vi "BRig_Host_dataRunState__entryAdd_v3.vi"(0 "input_dataPlot":u16[][](array[numeric]), 1 "input_dataTS":u16[][](array[numeric]), 2 "input_idx":i32[](array[numeric]), 4 "input_nTrial":u16, 5 "input_LorR":u16, 7 "input_sSelection":u16, 8 "input_trig_l2":u16, 9 "input_tSelection":u16, 10 "input_trig_l1":u16, 11 "input_tSelectionPlot":u16, 13 "input_iSelection":u16) -> (14 "output_dataPlot":u16[][](array[numeric]), 15 "output_dataTS":u16[][](array[numeric]), 16 "output_idx":i32[](array[numeric]), 18 "output_updatePlot":bool)   [LabVIEW 2014]
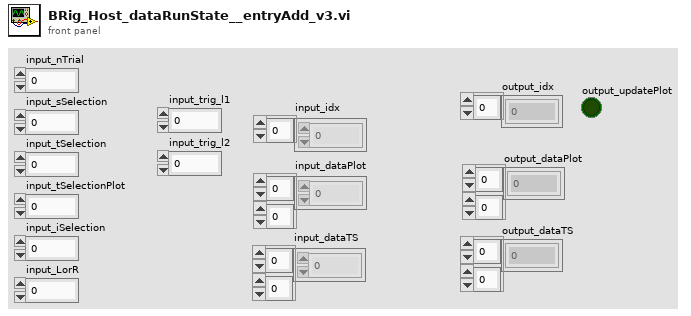
[diagram p1: front panel]
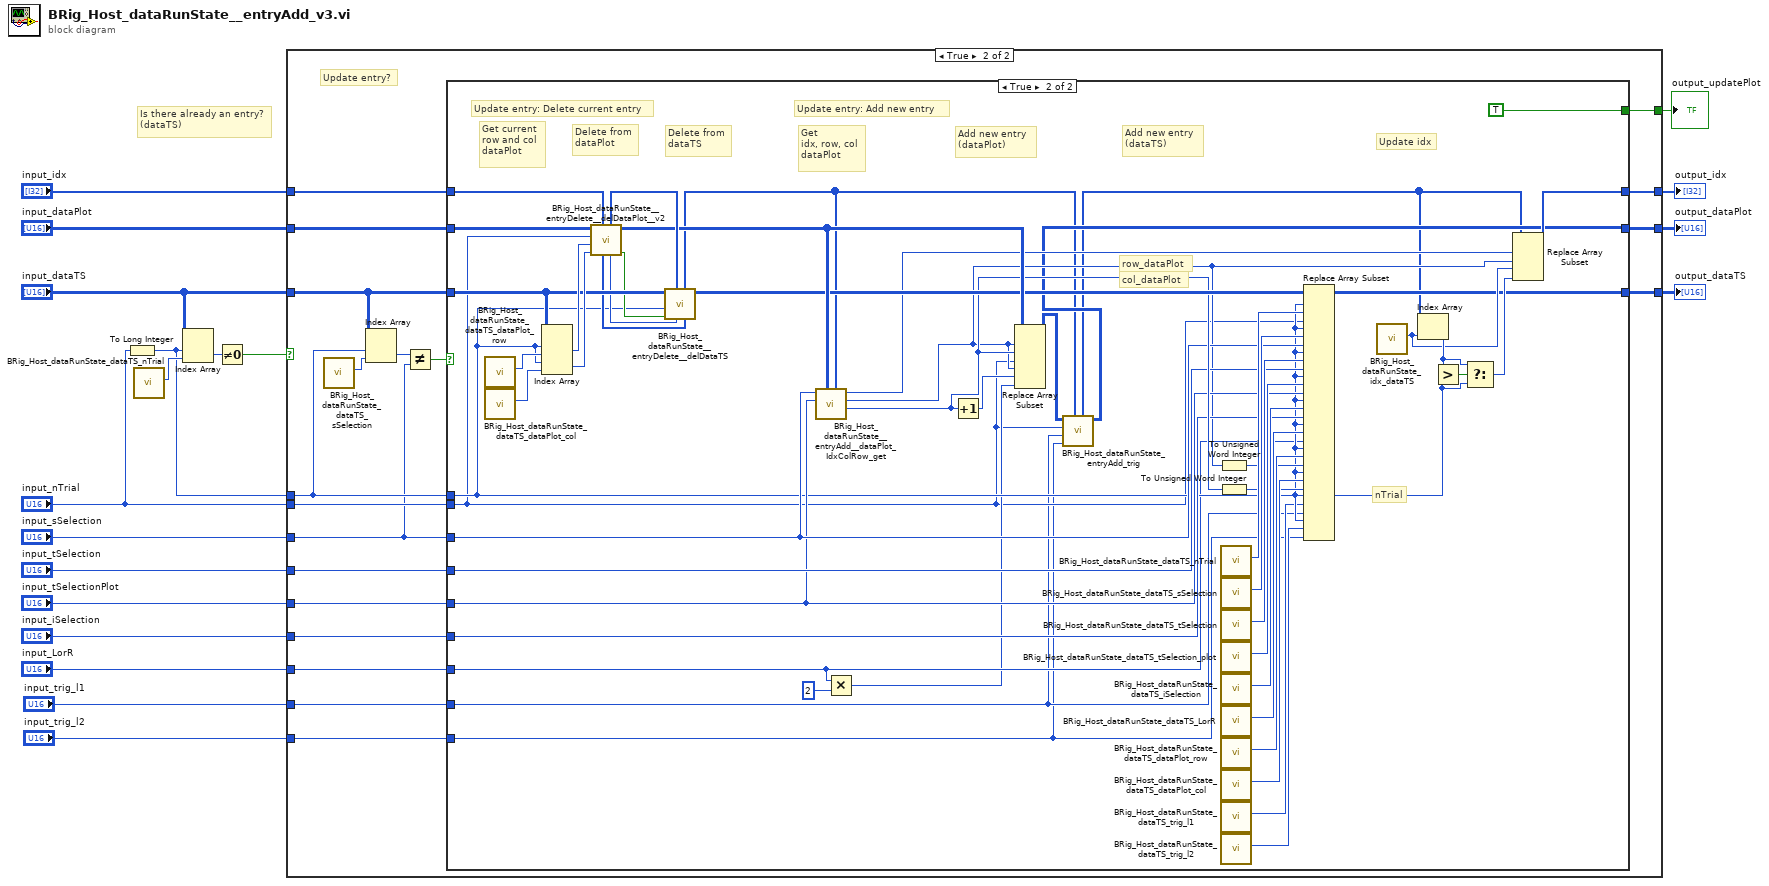
[diagram p0: block diagram]
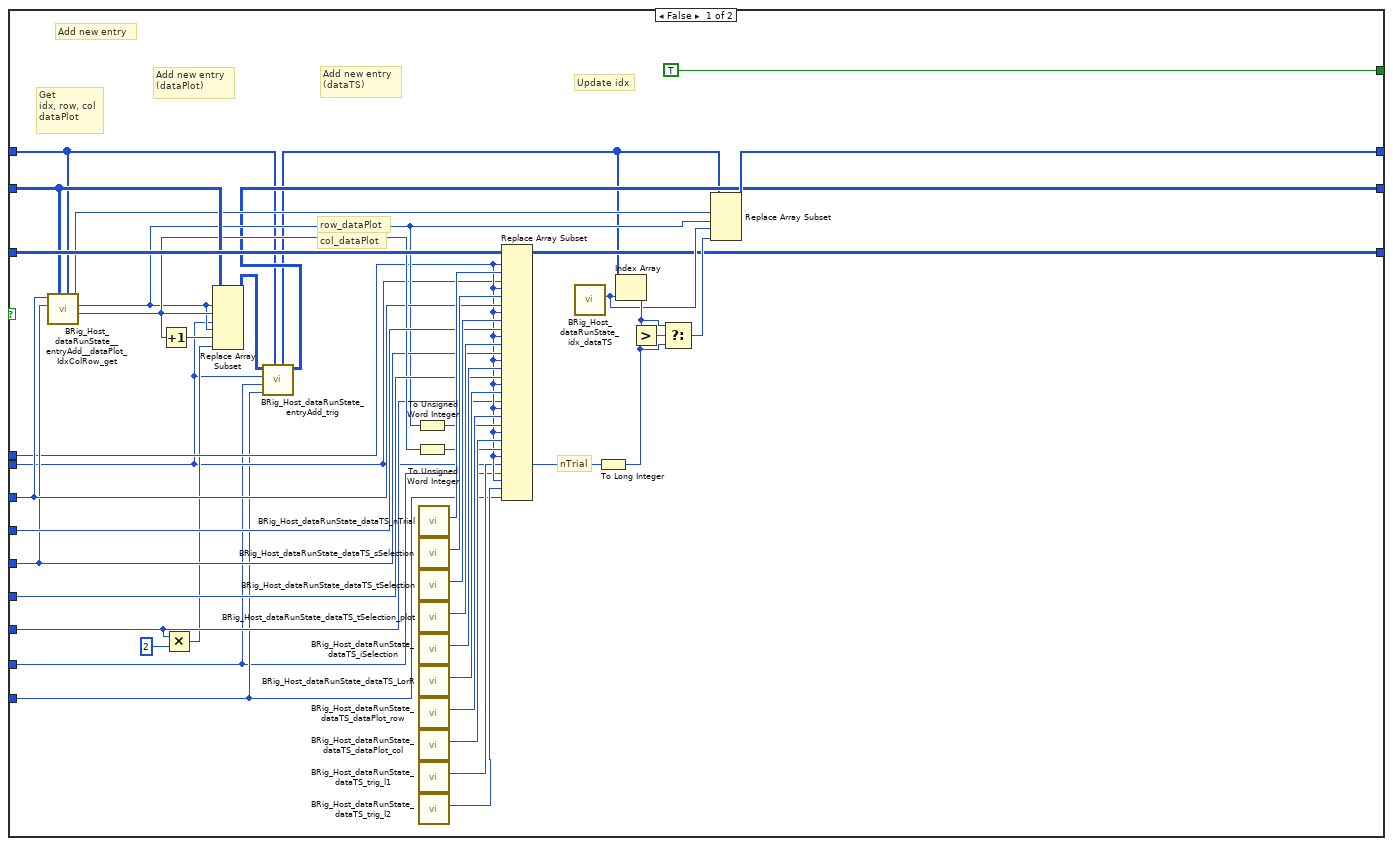
[diagram p2: hidden frame]
diagram:
  # "Is there already an entry?\n(dataTS)"
  n1 = To Long Integer(number="input_nTrial") -> (32bit integer=w15:i32)
  n2 = call "BRig_Host_dataRunState_dataTS_nTrial.vi"() -> ("output_idx_dataTS_nTrial"=w19:i32)  [unwired: 11 in]
  n3 = Index Array(array="input_dataTS", index (row)=w15, index (col)=w19) -> (element=w18:u16)
  n4 = Not Equal To 0?(x=w18) -> (x != 0?=w17:bool)
  n5 = case shown="True" w17 {
    tunnel: "input_nTrial" -> [w22 w69]
    tunnel: w15 -> [w31 w71]
    tunnel: "input_dataTS" -> [w60 w73]
    tunnel: "input_idx" -> [w24 w77]
    tunnel: "input_dataPlot" -> [w38 w75]
    tunnel: "input_sSelection" -> [w35 w63]
    tunnel: "input_tSelectionPlot" -> [w34 w70]
    tunnel: "input_iSelection" -> [w48 w66]
    tunnel: "input_LorR" -> [w28 w68]
    tunnel: [w50 w76] -> w6
    tunnel: [w25 w74] -> w5
    tunnel: [w43 w72] -> w4
    tunnel: "input_tSelection" -> [w49 w67]
    tunnel: [TRUE w65] -> w3
    tunnel: "input_trig_l1" -> [w20 w62]
    tunnel: "input_trig_l2" -> [w21 w61]
    frame False {
      # "Get\nidx, row, col\ndataPlot"
      # "nTrial"
      # "row_dataPlot"
      # "col_dataPlot"
      # "Update idx"
      # "Add new entry\n(dataPlot)"
      # "Add new entry"
      # "Add new entry\n(dataTS)"
      n6 = call "BRig_Host_dataRunState__entryAdd__dataPlot_IdxColRow_get.vi"("input_idx"=w24, "input_dataPlot"=w38, "input_tSelectionPlot"=w34, "input_sSelection"=w35) -> ("output_col_dataPlot"=w36:i32, "output_row_dataPlot"=w33:i32, "output_idx_dataPlot"=w37:i32)  [unwired: 5 in]
      n7 = Increment(x=w36) -> (x+1=w51:i32)
      n8 = Multiply(x=w28, y=u16 2) -> (x*y=w27:u16)
      n9 = Replace Array Subset(array=w38, new element #1=w22, index (row) #1=w33, index (col) #1=w36, new element #2=w27, index (row) #2=w33, index (col) #2=w51) -> (w26:u16[][])
      n10 = call "BRig_Host_dataRunState_entryAdd_trig.vi"("input_idx"=w24, "input_trig_l2"=w21, "input_trig_l1"=w20, "input_nTrial"=w22, "input_dataPlot"=w26) -> ("output_dataPlot"=w25:u16[][], "output_idx"=w23:i32[])  [unwired: 5 in]
      n11 = To Unsigned Word Integer(number=w33) -> (unsigned 16bit integer=w42:u16)
      n12 = To Unsigned Word Integer(number=w36) -> (unsigned 16bit integer=w41:u16)
      n13 = call "BRig_Host_dataRunState_dataTS_nTrial.vi"() -> ("output_idx_dataTS_nTrial"=w59:i32)  [unwired: 11 in]
      n14 = call "BRig_Host_dataRunState_dataTS_sSelection.vi"() -> ("output_idx_dataTS_sSelection"=w58:i32)  [unwired: 11 in]
      n15 = call "BRig_Host_dataRunState_dataTS_tSelection.vi"() -> ("output_idx_dataTS_tSelection"=w57:i32)  [unwired: 11 in]
      n16 = call "BRig_Host_dataRunState_dataTS_tSelection_plot.vi"() -> ("output_idx_dataTS_tSelection_plot"=w56:i32)  [unwired: 11 in]
      n17 = call "BRig_Host_dataRunState_dataTS_iSelection.vi"() -> ("output_idx_dataTS_iSelection"=w55:i32)  [unwired: 11 in]
      n18 = call "BRig_Host_dataRunState_dataTS_LorR.vi"() -> ("output_idx_dataTS_LorR"=w54:i32)  [unwired: 11 in]
      n19 = call "BRig_Host_dataRunState_dataTS_dataPlot_row.vi"() -> ("output_idx_dataTS_dataPlot_row"=w53:i32)  [unwired: 11 in]
      n20 = call "BRig_Host_dataRunState_dataTS_dataPlot_col.vi"() -> ("output_idx_dataTS_dataPlot_col"=w52:i32)  [unwired: 11 in]
      n21 = call "BRig_Host_dataRunState_dataTS_trig_l1.vi"() -> ("output_idx_dataTS_trig_l1"=w30:i32)  [unwired: 11 in]
      n22 = call "BRig_Host_dataRunState_dataTS_trig_l2.vi"() -> ("output_idx_dataTS_trig_l2"=w29:i32)  [unwired: 11 in]
      n23 = Replace Array Subset(array=w60, new element #1=w22, index (row) #1=w31, index (col) #1=w59, new element #2=w35, index (row) #2=w31, index (col) #2=w58, new element #3=w49, index (row) #3=w31, index (col) #3=w57, new element #4=w34, index (row) #4=w31, index (col) #4=w56, new element #5=w48, index (row) #5=w31, index (col) #5=w55, new element #6=w28, index (row) #6=w31, index (col) #6=w54, new element #7=w42, index (row) #7=w31, index (col) #7=w53, new element #8=w41, index (row) #8=w31, index (col) #8=w52, new element #9=w20, index (row) #9=w31, index (col) #9=w30, new element #10=w21, index (row) #10=w31, index (col) #10=w29) -> (w43:u16[][])
      n24 = call "BRig_Host_dataRunState_idx_dataTS.vi"() -> ("output_idx_dataTS"=w45:i32)  [unwired: 11 in]
      n25 = To Long Integer(number=w22) -> (32bit integer=w40:i32)
      n26 = Index Array(array=w23, index=w45) -> (element=w46:i32)
      n27 = Greater?(x=w46, y=w40) -> (0:w47:bool)
      n28 = Select(t=w46, s=w47, f=w40) -> (s? t:f=w44:i32)
      n29 = Replace Array Subset(array=w23, new element #1=w33, index #1=w37, new element #2=w44, index #2=w45) -> (w50:i32[])
    }
    frame True {
      # "Update entry?"
      n30 = call "BRig_Host_dataRunState_dataTS_sSelection.vi"() -> ("output_idx_dataTS_sSelection"=w64:i32)  [unwired: 11 in]
      n31 = Index Array(array=w73, index (row)=w71, index (col)=w64) -> (element=w79:u16)
      n32 = Not Equal?(x=w79, y=w63) -> (x != y?=w78:bool)
      n33 = case shown="True" w78 {
        tunnel: w77 -> [w82 w128]
        tunnel: [w82 w107] -> w76
        tunnel: w75 -> [w81 w131]
        tunnel: [w81 w88] -> w74
        tunnel: w73 -> [w80 w127]
        tunnel: [w80 w104] -> w72
        tunnel: w71 -> [_ w95]
        tunnel: w63 -> [_ w101]
        tunnel: w70 -> [_ w99]
        tunnel: w69 -> [_ w87]
        tunnel: w68 -> [_ w91]
        tunnel: w67 -> [_ w100]
        tunnel: w66 -> [_ w98]
        tunnel: [_ TRUE] -> w65
        tunnel: w62 -> [_ w86]
        tunnel: w61 -> [_ w85]
        frame False {
          # "Do nothing"
        }
        frame True {
          # "nTrial"
          # "row_dataPlot"
          # "col_dataPlot"
          # "Update idx"
          # "Add new entry\n(dataPlot)"
          # "Add new entry\n(dataTS)"
          # "Get\nidx, row, col\ndataPlot"
          # "Update entry: Add new entry"
          # "Delete from\ndataTS"
          # "Delete from\ndataPlot"
          # "Get current\nrow and col\ndataPlot"
          # "Update entry: Delete current entry"
          n34 = call "BRig_Host_dataRunState_dataTS_dataPlot_row.vi"() -> ("output_idx_dataTS_dataPlot_row"=w133:i32)  [unwired: 11 in]
          n35 = call "BRig_Host_dataRunState_dataTS_dataPlot_col.vi"() -> ("output_idx_dataTS_dataPlot_col"=w132:i32)  [unwired: 11 in]
          n36 = Index Array(array=w127, index (row) #1=w95, index (col) #1=w133, index (row) #2=w95, index (col) #2=w132) -> (element #1=w129:u16, element #2=w130:u16)
          n37 = call "BRig_Host_dataRunState__entryDelete__delDataPlot__v2.vi"("input_idx"=w128, "input_col_dataPlot"=w130, "input_row_dataPlot"=w129, "input_nTrial"=w87, "input_dataPlot"=w131) -> (0:"output_arrTrials"=w125:bool, "output_dataPlot"=w106:u16[][], "output_arrTrials_length"=w124:i32, "output_idx"=w126:i32[], 6:"output_arrTrials"=w123:i32[])  [unwired: 2 in]
          n38 = call "BRig_Host_dataRunState__entryDelete__delDataTS.vi"(4:"output_arrTrials"=w123, "output_arrTrials_length"=w124, "input_idx"=w126, 8:"output_arrTrials"=w125, "input_nTrial"=w95, "input_dataTS"=w127) -> ("output_dataTS"=w105:u16[][], "output_idx"=w84:i32[])  [unwired: 4 in]
          n39 = call "BRig_Host_dataRunState__entryAdd__dataPlot_IdxColRow_get.vi"("input_idx"=w84, "input_dataPlot"=w106, "input_tSelectionPlot"=w99, "input_sSelection"=w101) -> ("output_col_dataPlot"=w102:i32, "output_row_dataPlot"=w96:i32, "output_idx_dataPlot"=w103:i32)  [unwired: 5 in]
          n40 = Multiply(x=w91, y=u16 2) -> (x*y=w90:u16)
          n41 = Increment(x=w102) -> (x+1=w114:i32)
          n42 = Replace Array Subset(array=w106, new element #1=w87, index (row) #1=w96, index (col) #1=w102, new element #2=w90, index (row) #2=w96, index (col) #2=w114) -> (w89:u16[][])
          n43 = call "BRig_Host_dataRunState_entryAdd_trig.vi"("input_idx"=w84, "input_trig_l2"=w85, "input_trig_l1"=w86, "input_nTrial"=w87, "input_dataPlot"=w89) -> ("output_dataPlot"=w88:u16[][], "output_idx"=w83:i32[])  [unwired: 5 in]
          n44 = To Unsigned Word Integer(number=w96) -> (unsigned 16bit integer=w109:u16)
          n45 = To Unsigned Word Integer(number=w102) -> (unsigned 16bit integer=w108:u16)
          n46 = call "BRig_Host_dataRunState_dataTS_nTrial.vi"() -> ("output_idx_dataTS_nTrial"=w122:i32)  [unwired: 11 in]
          n47 = call "BRig_Host_dataRunState_dataTS_sSelection.vi"() -> ("output_idx_dataTS_sSelection"=w121:i32)  [unwired: 11 in]
          n48 = call "BRig_Host_dataRunState_dataTS_tSelection.vi"() -> ("output_idx_dataTS_tSelection"=w120:i32)  [unwired: 11 in]
          n49 = call "BRig_Host_dataRunState_dataTS_tSelection_plot.vi"() -> ("output_idx_dataTS_tSelection_plot"=w119:i32)  [unwired: 11 in]
          n50 = call "BRig_Host_dataRunState_dataTS_iSelection.vi"() -> ("output_idx_dataTS_iSelection"=w118:i32)  [unwired: 11 in]
          n51 = call "BRig_Host_dataRunState_dataTS_LorR.vi"() -> ("output_idx_dataTS_LorR"=w117:i32)  [unwired: 11 in]
          n52 = call "BRig_Host_dataRunState_dataTS_dataPlot_row.vi"() -> ("output_idx_dataTS_dataPlot_row"=w116:i32)  [unwired: 11 in]
          n53 = call "BRig_Host_dataRunState_dataTS_dataPlot_col.vi"() -> ("output_idx_dataTS_dataPlot_col"=w115:i32)  [unwired: 11 in]
          n54 = call "BRig_Host_dataRunState_dataTS_trig_l1.vi"() -> ("output_idx_dataTS_trig_l1"=w94:i32)  [unwired: 11 in]
          n55 = call "BRig_Host_dataRunState_dataTS_trig_l2.vi"() -> ("output_idx_dataTS_trig_l2"=w93:i32)  [unwired: 11 in]
          n56 = Replace Array Subset(array=w105, new element #1=w87, index (row) #1=w95, index (col) #1=w122, new element #2=w101, index (row) #2=w95, index (col) #2=w121, new element #3=w100, index (row) #3=w95, index (col) #3=w120, new element #4=w99, index (row) #4=w95, index (col) #4=w119, new element #5=w98, index (row) #5=w95, index (col) #5=w118, new element #6=w91, index (row) #6=w95, index (col) #6=w117, new element #7=w109, index (row) #7=w95, index (col) #7=w116, new element #8=w108, index (row) #8=w95, index (col) #8=w115, new element #9=w86, index (row) #9=w95, index (col) #9=w94, new element #10=w85, index (row) #10=w95, index (col) #10=w93) -> (w104:u16[][])
          n57 = call "BRig_Host_dataRunState_idx_dataTS.vi"() -> ("output_idx_dataTS"=w111:i32)  [unwired: 11 in]
          n58 = Index Array(array=w83, index=w111) -> (element=w112:i32)
          n59 = Greater?(x=w112, y=w95) -> (0:w113:bool)
          n60 = Select(t=w112, s=w113, f=w95) -> (s? t:f=w110:i32)
          n61 = Replace Array Subset(array=w83, new element #1=w96, index #1=w103, new element #2=w110, index #2=w111) -> (w107:i32[])
        }
      }
    }
  }
  "output_idx" <- w6
  "output_dataPlot" <- w5
  "output_dataTS" <- w4
  "output_updatePlot" <- w3
